vi "PULSE ON.vi"(9 "Pulse Length (ms)":u32=500, 10 "Input":bool) -> (2 "Output":bool)   [LabVIEW 2015]
doc: "The PULSE ON, when given a True input, will immediately output True for the specified delay, then output False. When the input reverts back to False, the pulse will reset, and emmit a pulse again when the input changes back to True."
panel:
  in  "Delay_TOF":T1={"Timer_States"=enum."Input_False_Timing", "Delay-Done_Time"=0}
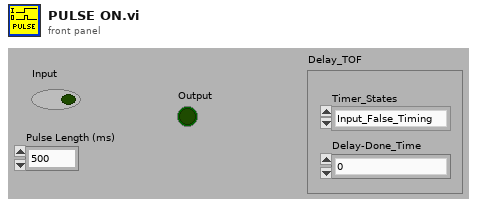
[diagram p1: front panel]
types:
  T1 = cluster{"Timer_States":enum16{"Input_True", "Input_False_Timing", "Input_False_Timing_Complete"}, "Delay-Done_Time":u32}
  T2 = enum16{"Input_True", "Input_False_Timing", "Input_False_Timing_Complete"}
  T3 = enum16{"Input_True", "Input_True_Timing", "Input_True_Timing_Complete"}
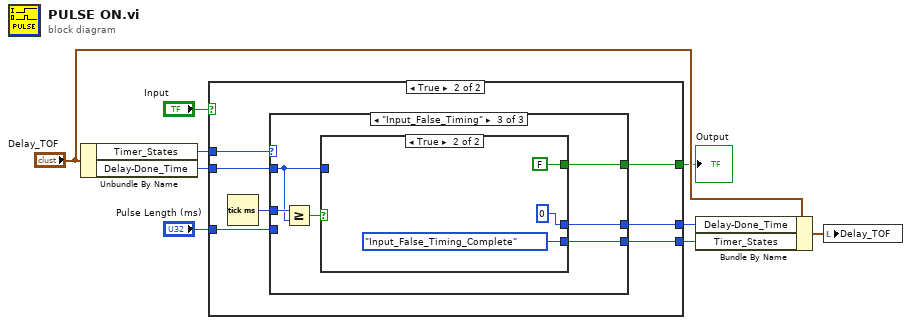
[diagram p0: block diagram]
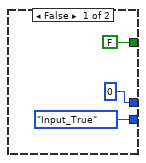
[diagram p2: hidden frame]
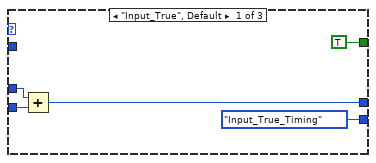
[diagram p3: hidden frame]
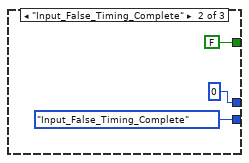
[diagram p4: hidden frame]
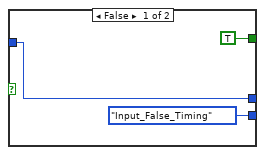
[diagram p5: hidden frame]
diagram:
  n1 = Unbundle By Name("Delay_TOF") -> ("Timer_States"=w5:T2, "Delay-Done_Time"=w8:u32)
  n2 = case shown="True" "Input" {
    tunnel: [FALSE w16] -> w1
    tunnel: [T2."Input_True" ("Timer_States") w17] -> w2
    tunnel: [u32 0 ("Delay-Done_Time") w18] -> w3
    tunnel: w8 -> [_ w13]
    tunnel: w5 -> [_ w15]
    tunnel: "Pulse Length (ms)" -> [_ w14]
    frame False {
    }
    frame True {
      n3 = Tick Count (ms)() -> (millisecond timer value=w19:u32)
      n4 = case shown="\"Input_False_Timing\"" w15 {
        tunnel: w19 -> [w23 _ w33]
        tunnel: [w21 u32 0 ("Delay-Done_Time") w28] -> w18
        tunnel: [T3."Input_True_Timing" ("Timer_States") T2."Input_False_Timing_Complete" ("Timer_States") w31] -> w17
        tunnel: [TRUE FALSE w30] -> w16
        tunnel: w14 -> [w22 _ _]
        tunnel: w13 -> [_ _ w29]
        frame "Input_True", Default {
          n5 = Add(x=w23, y=w22) -> (x+y=w21:u32)
        }
        frame "Input_False_Timing_Complete" {
        }
        frame "Input_False_Timing" {
          n6 = Greater Or Equal?(x=w33, y=w29) -> (x >= y?=w32:bool)
          n7 = case shown="True" w32 {
            tunnel: [T2."Input_False_Timing" ("Timer_States") T2."Input_False_Timing_Complete" ("Timer_States")] -> w31
            tunnel: [TRUE FALSE] -> w30
            tunnel: w29 -> [w34 _]
            tunnel: [w34 u32 0 ("Delay-Done_Time")] -> w28
            frame False {
            }
            frame True {
            }
          }
        }
      }
    }
  }
  "Output" <- w1
  n8 = Bundle By Name(cluster="Delay_TOF", "Delay-Done_Time"=w3, "Timer_States"=w2) -> (w7:T1)
  n9 = local write "Delay_TOF"(w7) -> ()
